vi "Dialog_Input.vi"(8 "error in (no error)":errorcluster, 11 "Caption.Text":string) -> (0 "error out":errorcluster, 2 "String out":string, 3 "true":bool)   [LabVIEW 2013]
panel:
  in  "String in":string caption="2"
  in  "OK Button":bool
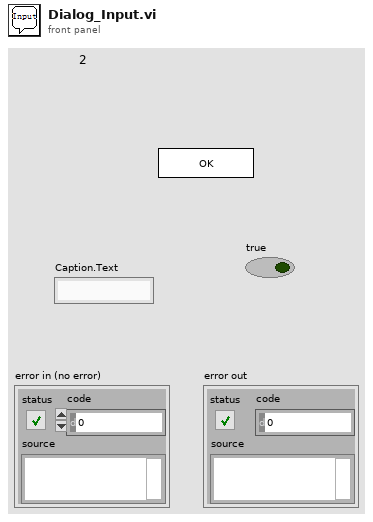
[diagram p1: front panel]
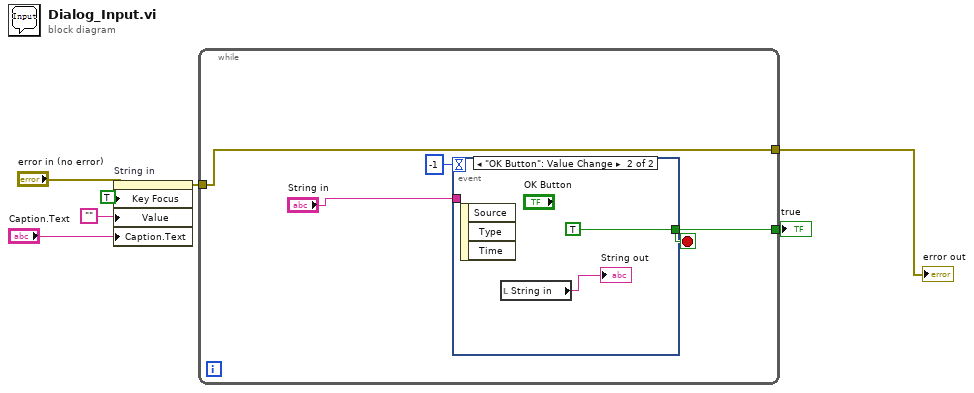
[diagram p0: block diagram]
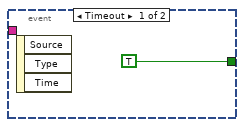
[diagram p2: hidden frame]
diagram:
  n1 = property on="String in" class="Str"(error in="error in (no error)", "Key Focus"=TRUE, "Value"="", "Caption.Text"="Caption.Text") -> (error out=w5:errorcluster)  [unwired: 1 in, 1 out]
  n2 = while {
    tunnel: [w11] -> w7
    tunnel: w5 -> [w9]
    tunnel: [w9] -> w2
    stop <- w11 stop-if-true
    n3 = event shown="[1] \"OK Button\": Value Change" {
      selector: _ -> [_ _]
      dyn-events: _ -> [_ _]
      timeout: -1 -> [_ _]
      tunnel: [TRUE TRUE] -> w11
      tunnel: "String in" -> [_ _]
      event Timeout {
        n4 = event-data() -> ()  [unwired: 1 in, 3 out]
      }
      event "OK Button": Value Change {
        n5 = event-data() -> ()  [unwired: 1 in, 3 out]
        n6 = local read "String in"() -> (→"String out":string)
      }
    }
  }
  "true" <- w7
  "error out" <- w2
